vi "Eval_MultiVar_SglRes.vi"(8 "error in (no error)":errorcluster, 9 "varValues":dbl[](array[numeric]) format="%#_13g", 10 "varNames":string[](array[string]), 11 "mupExpr in":refnum<data-value>) -> (0 "error out":errorcluster, 2 "Result":dbl format="%#_13g", 3 "mupExpr out":refnum<data-value>)   [LabVIEW 2015, in "mupExpr.lvclass"]
uses:
  mupExpr.lvclass
  mupExpr.lvclass/mupExpr.ctl
  mupLib/mupCheckError.vi
  mupLib/mupLibPath.vi
  mupLib/mupSetVarValue.vi
  <vilib>/Utility/error.llb/Error Cluster From Error Code.vi
  mupLib/mupLib.lvlib
panel:
  # "Update the value of multiple variables then evaluate the expression"
  # "If the variables are not found in the expression, an error will be generated"
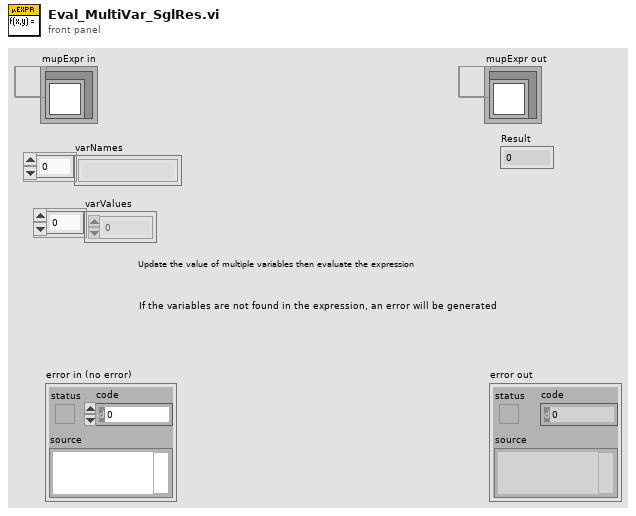
[diagram p1: front panel]
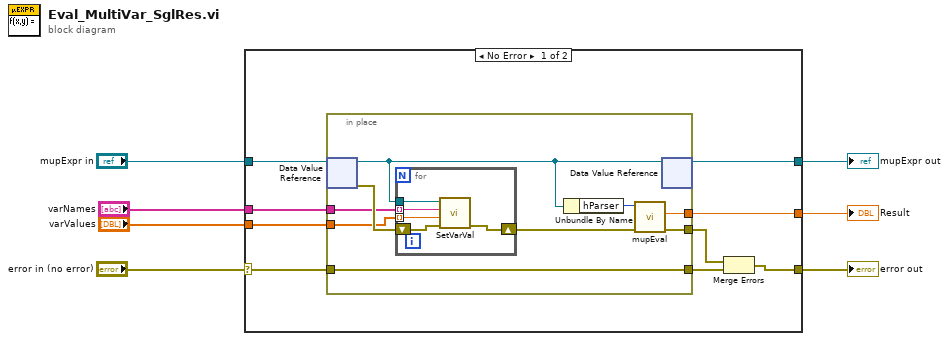
[diagram p0: block diagram]
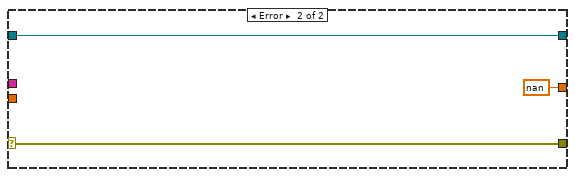
[diagram p2: hidden frame]
diagram:
  n1 = case shown="No Error" "error in (no error)" {
    selector: "error in (no error)" -> [w8 w33]
    tunnel: "varValues" -> [w16 _]
    tunnel: "varNames" -> [w15 _]
    tunnel: [w14 nan ("result")] -> w5
    tunnel: "mupExpr in" -> [w13 w31]
    tunnel: [w10 w33] -> w3
    tunnel: [w9 w31] -> w2
    frame No Error {
      n2 = in-place {
        in-place-border: w8 -> [w22]
        in-place-border: [w25] -> w11
        in-place-border: [w24] -> w14
        in-place-border: [w22] -> w12
        in-place-border: w16 -> [w19]
        in-place-border: w15 -> [w18]
        n3 = in-place-dvr #1(w13) -> (w17:refnum<class "mupExpr.lvclass">, w21:errorcluster)
        n4 = for {
          tunnel: w18 -> [w30] mode=indexing
          tunnel: w19 -> [w29] mode=indexing
          shift-right: [w27] -> w20
          shift-left: w21 -> [w28]
          tunnel: w17 -> [w26]
          n5 = call "SetVarVal.vi"("error in (no error)"=w28, "varValue"=w29, "varName"=w30, "muExpr in"=w26) -> ("error out"=w27:errorcluster)  [unwired: 6 in, 1 out]
        }
        n6 = Unbundle By Name(w17) -> ("hParser"=w23:u64)
        n7 = call "mupEval.vi"("error in (no error)"=w20, "hParser in"=w23) -> ("error out"=w25:errorcluster, "result"=w24:dbl)  [unwired: 7 in, 1 out]
        n8 = in-place-dvr #1(w17) -> (w9:refnum<data-value>)  [unwired: 1 out]
      }
      n9 = Merge Errors(w11, w12) -> (w10:errorcluster)
    }
    frame Error {
    }
  }
  "error out" <- w3
  "mupExpr out" <- w2
  "Result" <- w5
